vi "instrument_ring.vi"(4 "center":cluster{"x":i32, "y":i32}={"x"=51, "y"=51}, 5 "inside color":u32(colorbox), 6 "size":i16=44, 7 "ring color":u32(colorbox)=8016729, 10 "pict in":picture) -> (3 "new picture":picture)   [LabVIEW 2011]
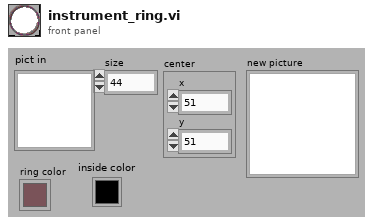
[diagram p1: front panel]
types:
  T1 = cluster{"Width":u16, "Style":enum32{"Solid", "Dash", "Dot", "DashDot", "DashDotDot"}}
  T2 = cluster{"[0]":dbl, "[1]":dbl, "[2]":dbl, "[3]":dbl}
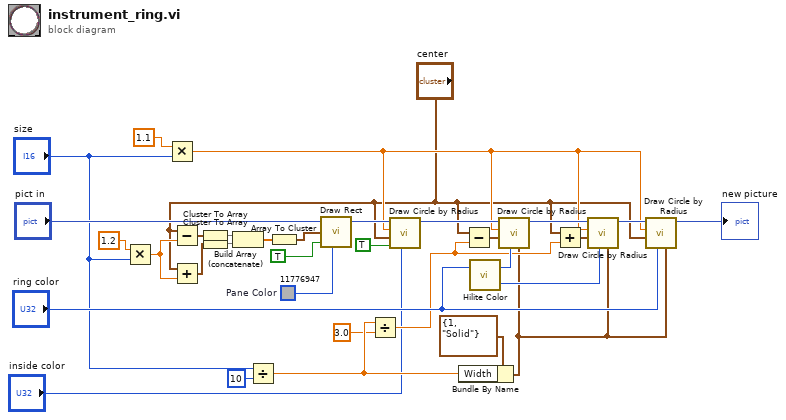
[diagram p0: block diagram]
diagram:
  w18 = u32 11776947  # Pane Color
  n1 = Multiply(x=1.2, y="size") -> (x*y=w7:dbl)
  n2 = Multiply(x=1.1, y="size") -> (x*y=w4:dbl)
  n3 = Subtract(x="center", y=w7) -> (x-y=w23:cluster{"x":dbl, "y":dbl})
  n4 = Add(x="center", y=w7) -> (x+y=w24:cluster{"x":dbl, "y":dbl})
  n5 = Cluster To Array(cluster=w23) -> (array=w21:dbl[])
  n6 = Cluster To Array(cluster=w24) -> (array=w22:dbl[])
  n7 = Build Array (concatenate)(w21, w22) -> (w20:dbl[])
  n8 = Divide(x="size", y=i16 10) -> (x/y=w14:dbl)
  n9 = Array To Cluster(array=w20) -> (cluster=w19:T2)
  n10 = call <vilib>:"Draw Rect.vi"("picture"="pict in", "rect"=w19, "fill?(F)"=TRUE, "color(black)"=w18) -> ("new picture"=w6:picture)  [unwired: 5 in]
  n11 = Divide(x=w14, y=3.0 ("y 2")) -> (x/y=w12:dbl)
  n12 = call <vilib>:"Draw Circle by Radius.vi"("color(black)"="inside color", "fill?(F)"=TRUE, "pixel center"="center", "radius"=w4, "picture"=w6) -> ("new picture"=w5:picture)  [unwired: 6 in]
  n13 = Bundle By Name(cluster=T1 {"Width"=1, "Style"=enum."Solid"} ("pen"), "Width"=w14) -> (w11:T1)
  n14 = Subtract(x="center", y=w12) -> (x-y=w27:cluster{"x":dbl, "y":dbl})
  n15 = call <vilib>:"Hilite Color.vi"("Color In"="ring color") -> ("Shadow"=w30:u32, "Hilite"=w29:u32)  [unwired: 1 in]
  n16 = call <vilib>:"Draw Circle by Radius.vi"("pen"=w11, "color(black)"=w29, "pixel center"=w27, "radius"=w4, "picture"=w5) -> ("new picture"=w28:picture)  [unwired: 6 in]
  n17 = Add(x="center", y=w12) -> (x+y=w26:cluster{"x":dbl, "y":dbl})
  n18 = call <vilib>:"Draw Circle by Radius.vi"("pen"=w11, "color(black)"=w30, "pixel center"=w26, "radius"=w4, "picture"=w28) -> ("new picture"=w31:picture)  [unwired: 6 in]
  n19 = call <vilib>:"Draw Circle by Radius.vi"("pen"=w11, "color(black)"="ring color", "pixel center"="center", "radius"=w4, "picture"=w31) -> ("new picture"=→"new picture":picture)  [unwired: 6 in]
